vi "Write # of charges.vi"(8 "error in (no error)":errorcluster, 10 "# of charges":i32, 11 "Particle Properties in":refnum<class "Particle Properties.lvclass">) -> (0 "error out":errorcluster, 3 "Particle Properties out":refnum<class "Particle Properties.lvclass">)   [LabVIEW 2014, in "Particle Properties.lvclass"]
uses:
  Particle Properties.lvclass
  Particle Properties.lvclass/Particle Properties.ctl
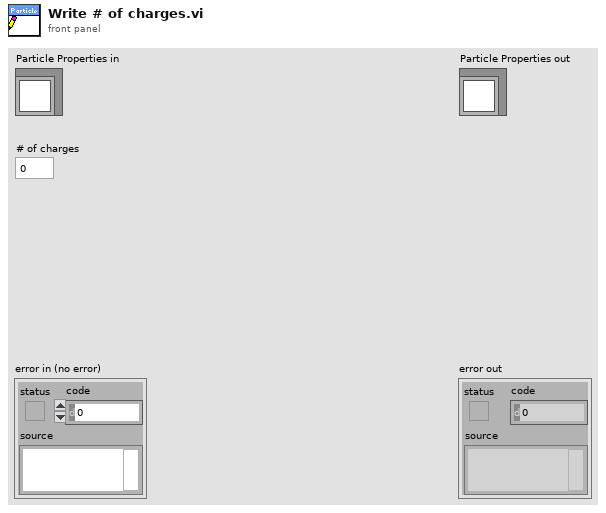
[diagram p1: front panel]
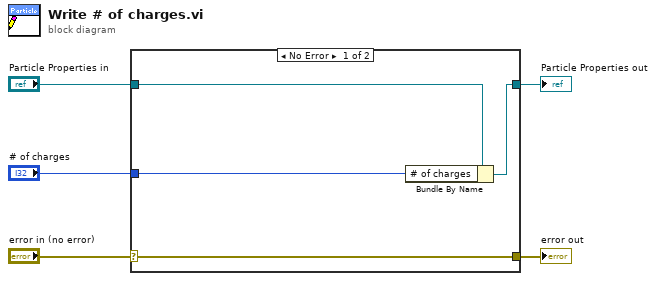
[diagram p0: block diagram]
diagram:
  n1 = case shown="No Error" "error in (no error)" {
    selector: "error in (no error)" -> [w9 w10]
    tunnel: [w9 w10] -> w4
    tunnel: [w7 w11] -> w2
    tunnel: "Particle Properties in" -> [w8 w11]
    tunnel: "# of charges" -> [w6 _]
    frame No Error {
      n2 = Bundle By Name(cluster=w8, "# of charges"=w6) -> (w7:refnum<class "Particle Properties.lvclass">)
    }
    frame Error {
    }
  }
  "error out" <- w4
  "Particle Properties out" <- w2
